vi "Read Electrical_Properties.vi"(8 "error in (no error)":errorcluster, 11 "EVI 79 in":refnum<class "EVI 79.lvclass">) -> (0 "error out":errorcluster, 2 "Electrical_Properties":cluster{"V_max":dbl, "I_max":dbl}={"V_max"=24.0, "I_max"=0.5}, 3 "EVI 79 out":refnum<class "EVI 79.lvclass">)   [LabVIEW 2025, in "EVI 79.lvclass"]
uses:
  EVI 79.lvclass
  EVI 79.lvclass/EVI 79.ctl
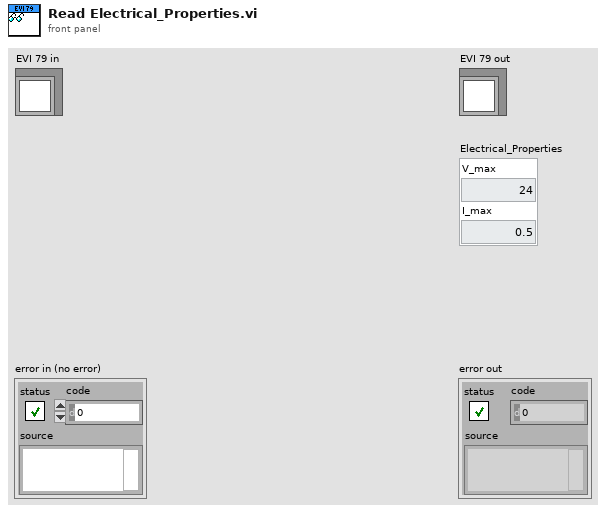
[diagram p1: front panel]
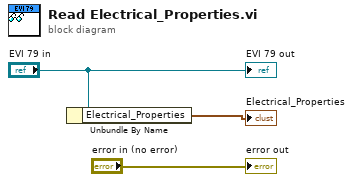
[diagram p0: block diagram]
diagram:
  n1 = Unbundle By Name("EVI 79 in") -> ("Electrical_Properties"=→"Electrical_Properties":cluster{"V_max":dbl, "I_max":dbl})
  "error out" <- "error in (no error)"
  "EVI 79 out" <- "EVI 79 in"
